vi "Actor Core.vi"(8 "Error In":errorcluster, 11 "CS++RTMainActor in":refnum<class "CS++RTMainActor.lvclass">) -> (0 "Error Out":errorcluster, 3 "Actor out":refnum<class "Actor.lvclass">)   [LabVIEW 2014, in "CS++RTMain.lvlib" / "CS++RTMainActor.lvclass"]
doc: "Initialize some shared variables and launch CS++RTWatchdogActor and Linked Network Actor.\n\n(<B>Filename</B>: Actor Framework.lvlib:Actor.lvclass:Actor Core.vi)\n\nReceives messages to the actor, reacts to them, and initiates any error handling that may shut the actor down.\n\nDescendant classes may override this VI to append parallel tasks for the actor to complete while it handles messages. Overrides use the Call Parent Method node."
uses:
  CS++RTMainActor.lvclass
  <vilib>/ActorFramework/Actor/Actor.lvclass
  <vilib>/NI/Actors/Linked Network Actor/Linked Network Actor/Linked Network Actor.lvclass
  CS++RTMainActor Messages/LNA Connection Status Msg/LNA Connection Status Msg.lvclass
  CS++RTWatchdog/CS++RTWatchdogActor.lvclass
  CS++RTMainActor Messages/LNA Return Message Msg/LNA Return Message Msg.lvclass
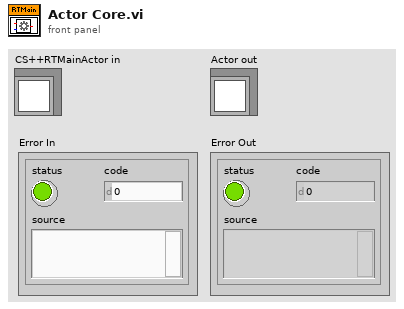
[diagram p1: front panel]
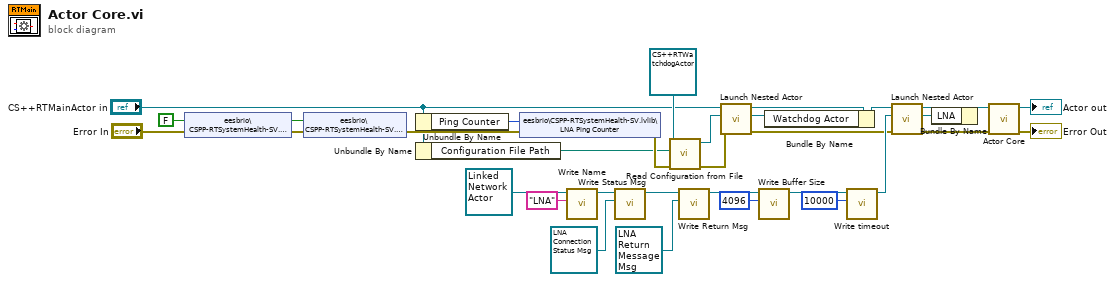
[diagram p0: block diagram]
diagram:
  w13 = FALSE
  n1 = shared-variable "eesbrio\\CSPP-RTSystemHealth-SV.lvlib\\LNA Reader"(w13, error in="Error In") -> (error out=w16:errorcluster)
  n2 = shared-variable "eesbrio\\CSPP-RTSystemHealth-SV.lvlib\\LNA Writer"(w13, error in=w16) -> (error out=w14:errorcluster)
  n3 = Unbundle By Name("CS++RTMainActor in") -> ("Ping Counter"=w17:u64)
  n4 = Unbundle By Name("CS++RTMainActor in") -> ("Configuration File Path"=w3:path)
  n5 = shared-variable "eesbrio\\CSPP-RTSystemHealth-SV.lvlib\\LNA Ping Counter"(w17, error in=w14) -> (error out=w6:errorcluster)
  n6 = call <vilib>:"Write Name.vi"("Name"="LNA", "Network Actor in"=refnum<class "Linked Network Actor.lvclass"> refnum ("Linked Network Actor.lvlib:Linked Network Actor.lvclass")) -> ("Network Actor out"=w24:refnum<class "Linked Network Actor.lvclass">)  [unwired: 9 in]
  n7 = call <vilib>:"Write Status Msg.vi"("Status Msg"=refnum<class "LNA Connection Status Msg.lvclass"> refnum ("CS++RTMain.lvlib:LNA Connection Status Msg.lvclass"), "Network Actor in"=w24) -> ("Network Actor out"=w25:refnum<class "Linked Network Actor.lvclass">)  [unwired: 9 in]
  n8 = call "Read Configuration from File.vi"("Error In"=w6, "Configuration File Path"=w3, "CS++RTWatchdogActor in"=refnum<class "CS++RTWatchdogActor.lvclass"> refnum ("CS++RTWatchdog.lvlib:CS++RTWatchdogActor.lvclass")) -> ("Error Out"=w8:errorcluster, "CS++RTWatchdogActor out"=w9:refnum<class "CS++RTWatchdogActor.lvclass">)  [unwired: 7 in]
  n9 = call <vilib>:"Write Return Msg.vi"("Return Msg"=refnum<class "LNA Return Message Msg.lvclass"> refnum ("CS++RTMain.lvlib:LNA Return Message Msg.lvclass"), "Linked Network Actor in"=w25) -> ("Linked Network Actor out"=w23:refnum<class "Linked Network Actor.lvclass">)  [unwired: 9 in]
  n10 = call <vilib>:"Launch Nested Actor.vi"("error in (no error)"=w8, "Nested Actor"=w9, "Caller Actor in"="CS++RTMainActor in") -> ("error out"=w5:errorcluster, "Nested Actor's Enqueuer"=w11:refnum<class "Message Enqueuer.lvclass">, "Caller Actor out"=w12:refnum<class "CS++RTMainActor.lvclass">)  [unwired: 6 in]
  n11 = call <vilib>:"Write Buffer Size.vi"("Buffer Size"=4096, "Network Actor in"=w23) -> ("Network Actor out"=w27:refnum<class "Linked Network Actor.lvclass">)  [unwired: 9 in]
  n12 = Bundle By Name(cluster=w12, "Watchdog Actor"=w11) -> (w7:refnum<class "CS++RTMainActor.lvclass">)
  n13 = call <vilib>:"Write timeout.vi"("timeout"=10000, "Network Actor in"=w27) -> ("Network Actor out"=w21:refnum<class "Linked Network Actor.lvclass">)  [unwired: 9 in]
  n14 = call <vilib>:"Launch Nested Actor.vi"("error in (no error)"=w5, "Nested Actor"=w21, "Caller Actor in"=w7) -> ("error out"=w22:errorcluster, "Nested Actor's Enqueuer"=w19:refnum<class "Message Enqueuer.lvclass">, "Caller Actor out"=w20:refnum<class "CS++RTMainActor.lvclass">)  [unwired: 6 in]
  n15 = Bundle By Name(cluster=w20, "LNA"=w19) -> (w18:refnum<class "CS++RTMainActor.lvclass">)
  n16 = call-parent "Actor Core.vi"("error in"=w22, "Actor in"=w18) -> ("error out"=→"Error Out":errorcluster, "Actor out"=→"Actor out":refnum<class "Actor.lvclass">)  [unwired: 8 in]
